vi "Write Multiple Properties.vi"(6 "timeout (ms)":i32=-1, 8 "error in (no error)":errorcluster, 9 "property_values":string[](array[string]), 10 "property_names":string[](array[string]), 11 "FlexLogger_gRPCAPI in":refnum<class "FlexLogger_gRPC.lvclass">) -> (0 "error out":errorcluster, 3 "FlexLogger_gRPCAPI out":refnum<class "FlexLogger_gRPC.lvclass">)   [LabVIEW 2020, in "FlexLogger_gRPC.lvlib" / "FlexLogger_gRPC.lvclass"]
doc: "Sets all test properties to currently opened project in flexlogger"
uses:
  FlexLogger_gRPC.lvclass
  FlexLogger_client/RPC Messages/flexlogger_SetTestPropertiesRequest.ctl
  FlexLogger_client/RPC Messages/flexlogger_ElementIdentifier.ctl
  FlexLogger_client/RPC Messages/flexlogger_TestProperty.ctl
  FlexLogger_gRPC.lvclass/FlexLogger_gRPC.ctl
  FlexLogger_client/FlexLogger_client.lvlib
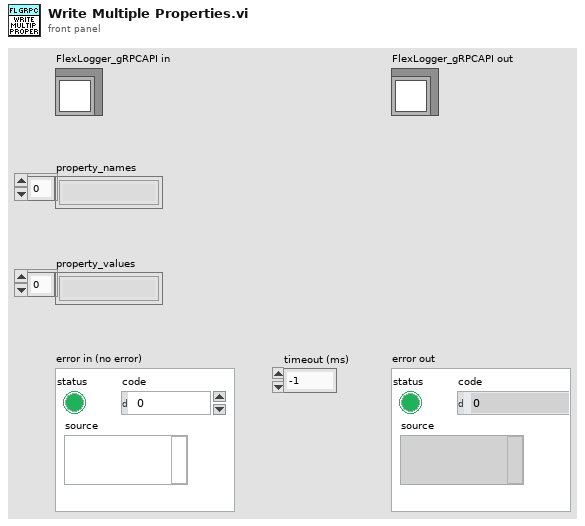
[diagram p1: front panel]
types:
  T1 = typedef "FlexLogger_client.lvlib/flexlogger_SetTestPropertiesRequest.ctl" = cluster{"document_identifier":T2, "test_properties":T3[]}
  T2 = typedef "FlexLogger_client.lvlib/flexlogger_ElementIdentifier.ctl" = cluster{"project_id":string, "file_name":string, "element_id":string, "subpart_id":string}
  T3 = typedef "FlexLogger_client.lvlib/flexlogger_TestProperty.ctl" = cluster{"property_name":string, "property_value":string, "prompt_on_start":bool}
  T4 = typedef "grpc-lvsupport-release.lvlib/grpcId.ctl" = u64
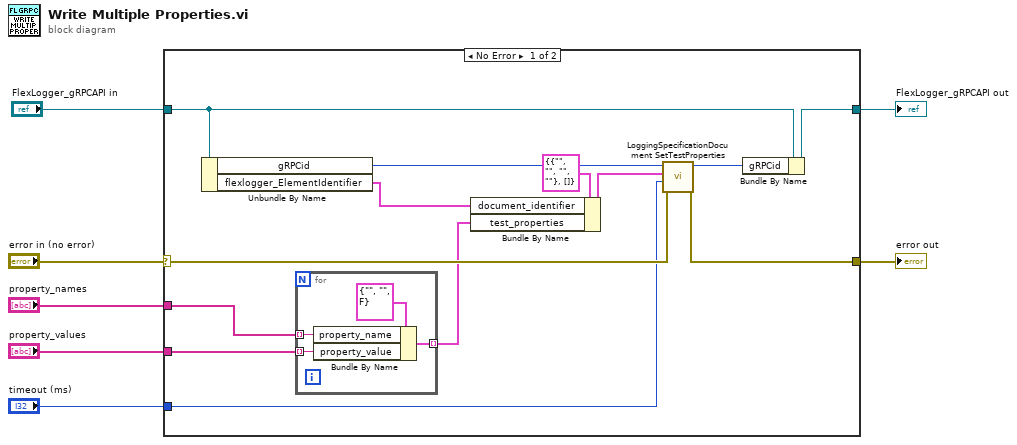
[diagram p0: block diagram]
diagram:
  n1 = case shown="No Error" "error in (no error)" {
    selector: "error in (no error)" -> [w16 w25]
    tunnel: "FlexLogger_gRPCAPI in" -> [w20 w26]
    tunnel: [w19 w26] -> w7
    tunnel: [w15 w25] -> w6
    tunnel: "timeout (ms)" -> [w14 _]
    tunnel: "property_names" -> [w10 _]
    tunnel: "property_values" -> [w9 _]
    frame No Error {
      n2 = Unbundle By Name(w20) -> ("gRPCid"=w18:T4, "flexlogger_ElementIdentifier"=w12:T2)
      n3 = for {
        tunnel: w10 -> [w23] mode=indexing
        tunnel: w9 -> [w22] mode=indexing
        tunnel: [w21] -> w8 mode=indexing
        n4 = Bundle By Name(cluster=T3 {"property_name"="", "property_value"="", "prompt_on_start"=FALSE} ("flexlogger_TestProperty"), "property_name"=w23, "property_value"=w22) -> (w21:T3)
      }
      n5 = Bundle By Name(cluster=T1 {"document_identifier"={"project_id"="", "file_name"="", "element_id"="", "subpart_id"=""}, "test_properties"=[]} ("Request Data"), "document_identifier"=w12, "test_properties"=w8) -> (w11:T1)
      n6 = call "LoggingSpecificationDocument SetTestProperties.vi"("error in"=w16, "timeout (ms)"=w14, "Request Data"=w11, "gRPC ID"=w18) -> ("error out"=w15:errorcluster, "gRPC ID out"=w17:T4)  [unwired: 5 in, 1 out]
      n7 = Bundle By Name(cluster=w20, "gRPCid"=w17) -> (w19:refnum<class "FlexLogger_gRPC.lvclass">)
    }
    frame Error {
    }
  }
  "error out" <- w6
  "FlexLogger_gRPCAPI out" <- w7
